vi "Verify Destination Path.vi"(8 "error in (no error)":errorcluster, 10 "Custom Device Name":string, 11 "Custom Device Path":path) -> (0 "error out":errorcluster)   [LabVIEW 2014, in "NIVS_ScriptedModuleTemplate_MetaDataObj.lvclass"]
uses:
  NIVS_ScriptedModuleTemplate_MetaDataObj.lvclass
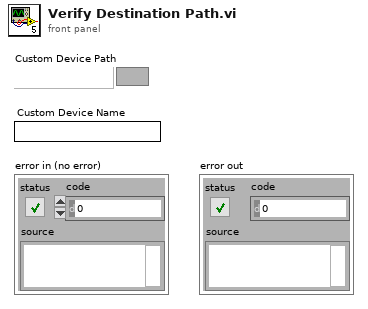
[diagram p1: front panel]
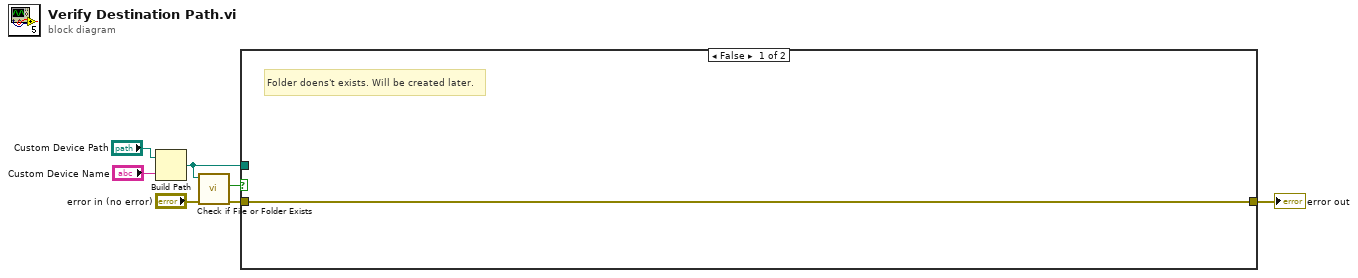
[diagram p0: block diagram]
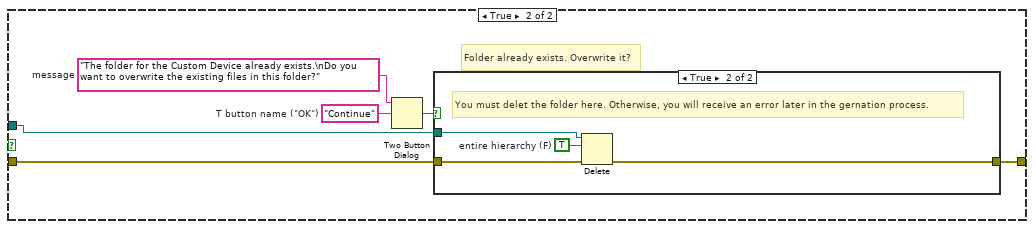
[diagram p2: hidden frame]
diagram:
  n1 = Build Path(base path="Custom Device Path", name or relative path="Custom Device Name") -> (appended path=w7:path)
  n2 = call <vilib>:"Check if File or Folder Exists.vi"("error in (no error)"="error in (no error)", "path"=w7) -> ("error out"=w5:errorcluster, "file or folder exists?"=w4:bool)  [unwired: 8 out]
  n3 = case shown="False" w4 {
    tunnel: w5 -> [w8 w11]
    tunnel: [w8 w10] -> w6
    tunnel: w7 -> [_ w9]
    frame False {
      # "Folder doens't exists. Will be created later."
    }
    frame True {
      w13 = "Continue"  # T button name ("OK")
      w14 = "The folder for the Custom Device already exists.\nDo you want to overwrite the existing files in this folder?"  # message
      # "Folder already exists. Overwrite it?"
      n4 = Two Button Dialog(message=w14, 2:w13) -> (T button?=w12:bool)  [unwired: 1 in]
      n5 = case shown="True" w12 {
        tunnel: w11 -> [w15 w19]
        tunnel: [w15 w18] -> w10
        tunnel: w9 -> [_ w17]
        frame False {
          # "Cancle"
        }
        frame True {
          w16 = TRUE  # entire hierarchy (F)
          # "You must delet the folder here. Otherwise, you will receive an error later in the gernation process."
          n6 = Delete(path (use dialog)=w17, entire hierarchy (F)=w16, error in=w19) -> (error out=w18:errorcluster)  [unwired: 2 in, 2 out]
        }
      }
    }
  }
  "error out" <- w6
